vi "aod_calc_amplitude.vi"(8 "FPGA parameters in":T1 {"AOD center frequ. (Hz)_y" format="%.14g"; "AOD half bandwidth_y" format="%.14g"; "AOD Bandwidth_y (Hz)" format="%_6f"; "AOD center frequ. (Hz)_x" format="%.14g"; "cos Phi" format="%.35g"; "sin Phi" format="%.35g"; "AOD_Scale_Factor (1/Zoom)" format="%.35g"; "AOD half bandwidth_x" format="%.14g"; "AOD Bandwidth_x (Hz)" format="%_6f"}, 9 "channel selector in":enum16{"x-channel", "y-channel"}(ring), 10 "amplitude compensation?":bool, 11 "scaled input":fxp<+/-,36,32> format="%.14g") -> (0 "FPGA parameters out":T1 {"AOD center frequ. (Hz)_y" format="%.14g"; "AOD half bandwidth_y" format="%.14g"; "AOD Bandwidth_y (Hz)" format="%_6f"; "AOD center frequ. (Hz)_x" format="%.14g"; "cos Phi" format="%.35g"; "sin Phi" format="%.35g"; "AOD_Scale_Factor (1/Zoom)" format="%.35g"; "AOD half bandwidth_x" format="%.14g"; "AOD Bandwidth_x (Hz)" format="%_6f"}, 3 "output":u16)   [LabVIEW 2010]
uses:
  FPGA_parameters_cluster.ctl
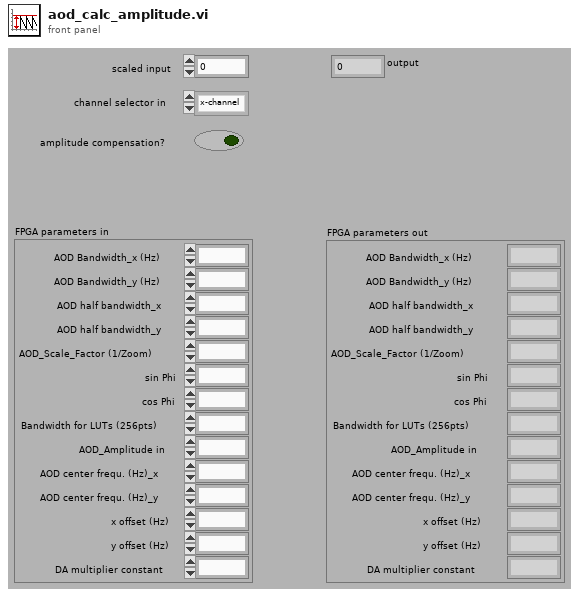
[diagram p1: front panel]
types:
  T1 = typedef "FPGA_parameters_cluster.ctl" = cluster{"AOD Bandwidth_x (Hz)":fxp<+,36,32>, "AOD Bandwidth_y (Hz)":fxp<+,36,32>, "AOD half bandwidth_x":fxp<+,36,32>, "AOD half bandwidth_y":fxp<+,36,32>, "AOD_Scale_Factor (1/Zoom)":fxp<+,36,2>, "sin Phi":fxp<+/-,36,2>, "cos Phi":fxp<+/-,36,2>, "Bandwidth for LUTs (256pts)":fxp<+,36,0>, "AOD_Amplitude in":u16, "AOD center frequ. (Hz)_x":fxp<+,36,32>, "AOD center frequ. (Hz)_y":fxp<+,36,32>, "x offset (Hz)":fxp<+/-,36,32>, "y offset (Hz)":fxp<+/-,36,32>, "DA multiplier constant":fxp<+,64,4>}
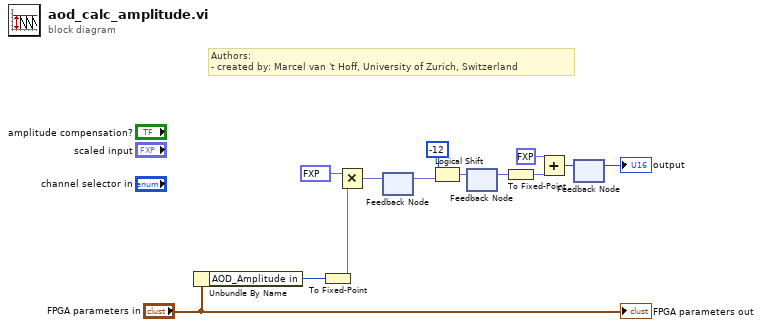
[diagram p0: block diagram]
diagram:
  # "Authors: \n- created by: Marcel van 't Hoff, University of Zurich, Switzerland"
  n1 = Unbundle By Name("FPGA parameters in") -> ("AOD_Amplitude in"=w3:u16)
  n2 = To Fixed-Point(number=w3) -> (fixed-point=w11:fxp<+,12,12>)  [unwired: 1 out]
  n3 = Multiply(x=fxp<+,12,12> 4095.0, y=w11) -> (x*y=w5:fxp<+,24,24>)
  n4 = feedback #1() -> (w4:fxp<+,24,24>)  [unwired: 1 out]
  n5 = feedback-in #1(w5) -> ()
  n6 = Logical Shift(y=i8 -12, x=w4) -> (x << y=w2:fxp<+,24,24>)
  n7 = feedback #2() -> (w1:fxp<+,24,24>)  [unwired: 1 out]
  n8 = feedback-in #2(w2) -> ()
  n9 = To Fixed-Point(number=w1) -> (fixed-point=w8:fxp<+,16,16>)  [unwired: 1 out]
  n10 = Add(x=fxp<+,2,2> 1.0, y=w8) -> (x+y=w7:u16)
  n11 = feedback-in #3(w7) -> ()
  n12 = feedback #3() -> (→"output":u16)  [unwired: 1 out]
  "FPGA parameters out" <- "FPGA parameters in"
